vi "slscswitch Close.vi"(8 "error in (no error)":errorcluster, 11 "SLSC Switch in":refnum<class "SLSC Switch.lvclass">) -> (0 "error out":errorcluster)   [LabVIEW 2015, in "SLSC Switch.lvclass"]
uses:
  SLSC Switch.lvclass
  SLSC Switch.lvclass/SLSC Switch.ctl
  <vilib>/SLSC/SLSC.lvlib
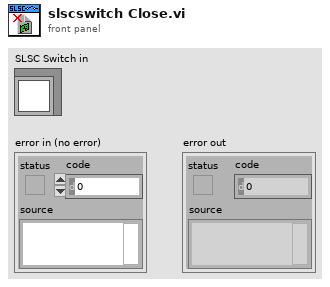
[diagram p1: front panel]
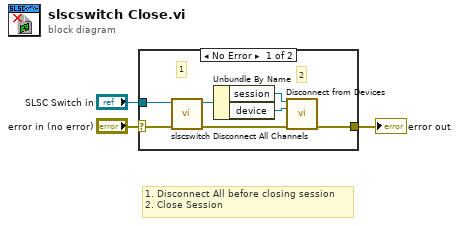
[diagram p0: block diagram]
diagram:
  # "1. Disconnect All before closing session\n2. Close Session"
  n1 = case shown="No Error" "error in (no error)" {
    selector: "error in (no error)" -> [w6 w11]
    tunnel: [w8 w11] -> w2
    tunnel: "SLSC Switch in" -> [w7 _]
    frame No Error {
      # "2"
      # "1"
      n2 = call "slscswitch Disconnect All Channels.vi"("error in (no error)"=w6, "SLSC Switch in"=w7) -> ("error out"=w5:errorcluster, "SLSC Switch out"=w4:refnum<class "SLSC Switch.lvclass">)  [unwired: 8 in]
      n3 = Unbundle By Name(w4) -> ("session"=w10:refnum<k21>, "device"=w9:refnum<k21>)
      n4 = call <vilib>:"Disconnect from Devices.vi"("session in"=w10, "devices"=w9, "error in (no error)"=w5) -> ("error out"=w8:errorcluster)  [unwired: 11 in, 1 out]
    }
    frame Error {
    }
  }
  "error out" <- w2
